vi "Result.vi"(8 "error in (no error)":errorcluster, 11 "IV_data in":refnum<class "IV_data.lvclass">) -> (0 "error out":errorcluster, 3 "IV_data out":refnum<class "IV_data.lvclass">)   [LabVIEW 2018, in "IV_data.lvclass"]
uses:
  IV_data.lvclass
  Abstract/Data/Data2D/Data2D.lvclass
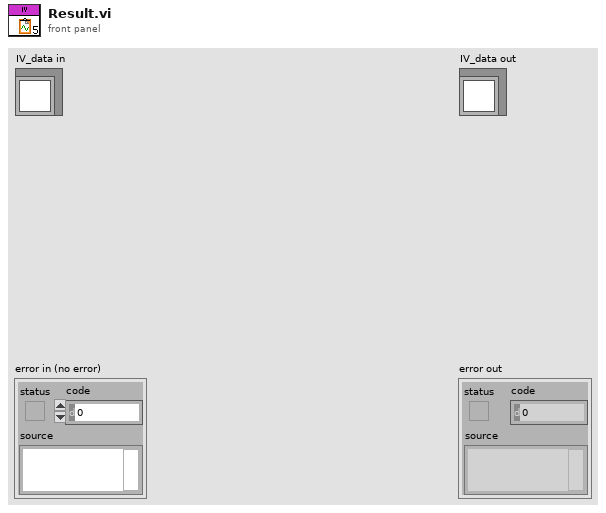
[diagram p1: front panel]
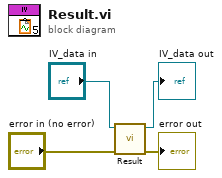
[diagram p0: block diagram]
diagram:
  n1 = call-parent "Result.vi"("error in (no error)"="error in (no error)", "Data2D in"="IV_data in") -> ("error out"=→"error out":errorcluster, "Data2D out"=→"IV_data out":refnum<class "IV_data.lvclass">)  [unwired: 8 in]
